vi "Graphics-Init Y-axis Overlay.vi"(0 "Ctl Refnum":refnum<vi>, 7 "Y-axis slider":refnum<vi>, 11 "error in (no error)":errorcluster) -> (15 "error out":errorcluster)   [LabVIEW 2020]
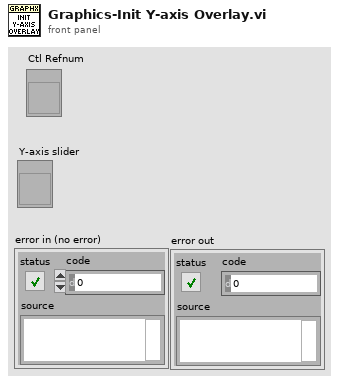
[diagram p1: front panel]
types:
  T1 = typedef "LVRectTypeDef.ctl" = cluster{"Left":i16, "Top":i16, "Right":i16, "Bottom":i16}
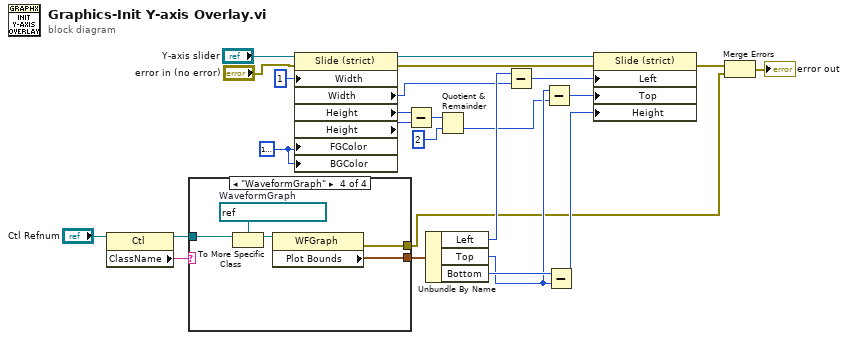
[diagram p0: block diagram]
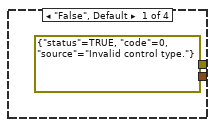
[diagram p2: hidden frame]
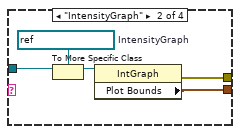
[diagram p3: hidden frame]
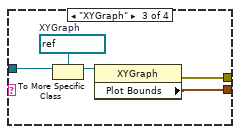
[diagram p4: hidden frame]
diagram:
  w4 = u32 16777216
  n1 = property class="Ctl"(reference="Ctl Refnum") -> (reference out=w1:refnum<vi>, "ClassName"=w2:string)  [unwired: 1 in, 1 out]
  n2 = case shown="\"WaveformGraph\"" w2 {
    tunnel: [_ w31 w36 w41] -> w20
    tunnel: [errorcluster {"status"=TRUE, "code"=0, "source"="Invalid control type."} ("error out") w30 w35 w40] -> w6
    tunnel: w1 -> [_ w29 w34 w39]
    frame "False", Default {
    }
    frame "IntensityGraph" {
      w28 = refnum<vi> refnum  # IntensityGraph
      n3 = To More Specific Class(target class=w28, reference=w29) -> (specific class reference=w27:refnum<vi>)  [unwired: 1 in, 1 out]
      n4 = property class="IntGraph"(reference=w27) -> (error out=w30:errorcluster, "Plot Bounds"=w31:T1)  [unwired: 1 in, 1 out]
    }
    frame "XYGraph" {
      w33 = refnum<vi> refnum  # XYGraph
      n5 = To More Specific Class(target class=w33, reference=w34) -> (specific class reference=w32:refnum<vi>)  [unwired: 1 in, 1 out]
      n6 = property class="XYGraph"(reference=w32) -> (error out=w35:errorcluster, "Plot Bounds"=w36:T1)  [unwired: 1 in, 1 out]
    }
    frame "WaveformGraph" {
      w38 = refnum<vi> refnum  # WaveformGraph
      n7 = To More Specific Class(target class=w38, reference=w39) -> (specific class reference=w37:refnum<vi>)  [unwired: 1 in, 1 out]
      n8 = property class="WFGraph"(reference=w37) -> (error out=w40:errorcluster, "Plot Bounds"=w41:T1)  [unwired: 1 in, 1 out]
    }
  }
  n9 = property class="Slide (strict)"(reference="Y-axis slider", error in="error in (no error)", "Width"=u32 1 ("Housing Size:Width"), "FGColor"=w4, "BGColor"=w4) -> (reference out=w23:refnum<vi>, error out=w18:errorcluster, "Width"=w16:u32, "Height"=w15:u32, "Height"=w14:u32)
  n10 = Subtract(x=w15, y=w14) -> (x-y=w13:u32)
  n11 = Unbundle By Name(w20) -> ("Left"=w21:i16, "Top"=w10:i16, "Bottom"=w24:i16)
  n12 = Quotient & Remainder(x=w13, y=u32 2) -> (floor(x/y)=w9:u32)  [unwired: 1 out]
  n13 = Subtract(x=w21, y=w16) -> (x-y=w22:u32)
  n14 = Subtract(x=w10, y=w9) -> (x-y=w11:u32)
  n15 = Subtract(x=w24, y=w10) -> (x-y=w25:i16)
  n16 = property class="Slide (strict)"(reference=w23, error in=w18, "Left"=w22, "Top"=w11, "Height"=w25) -> (error out=w8:errorcluster)  [unwired: 1 out]
  n17 = Merge Errors(w8, w6) -> (→"error out":errorcluster)
